vi "Poll Syringe-Line Valve Control.vi"(8 "error in (no error)":errorcluster, 11 "Syringe Line in":refnum<class "Syringe Line.lvclass">) -> ()   [LabVIEW 2015, in "cRIO-Carbondioxide.lvlib" / "CO2-Actor.lvlib" / "Syringe Line.lvclass"]
uses:
  Syringe Line.lvclass
  Syringe Line.lvclass/Syringe Line.ctl
  <vilib>/ActorFramework/Actor/Actor.lvclass/Actor.ctl
  <vilib>/ActorFramework/Message Enqueuer/Message Enqueuer.lvclass/Message Enqueuer.ctl
  Syringe Line Messages/Set Syringe Valve/Set Valve Msg/Set Syringe Valve Msg.lvclass/Set Syringe Valve Msg.ctl
  <vilib>/ActorFramework/Actor/Read Self Enqueuer.vi
  <vilib>/ActorFramework/Message Enqueuer/Enqueue.vi
  <vilib>/ActorFramework/Message Enqueuer/Init from Existing Queue.vi
  <vilib>/ActorFramework/Message Priority Queue/Priority Enqueue.vi
  <vilib>/ActorFramework/Actor/Actor.lvclass
  <vilib>/ActorFramework/Message Enqueuer/Message Enqueuer.lvclass
  Syringe Line Messages/Set Syringe Valve/Set Valve Msg/Set Syringe Valve Msg.lvclass
  cRIO-CO2/cRIO-CO2.lvclass
  CO2 Actor/CO2 Actor.lvclass
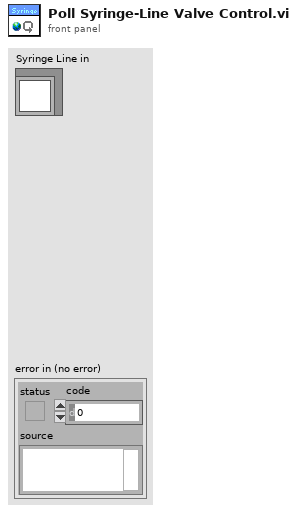
[diagram p1: front panel]
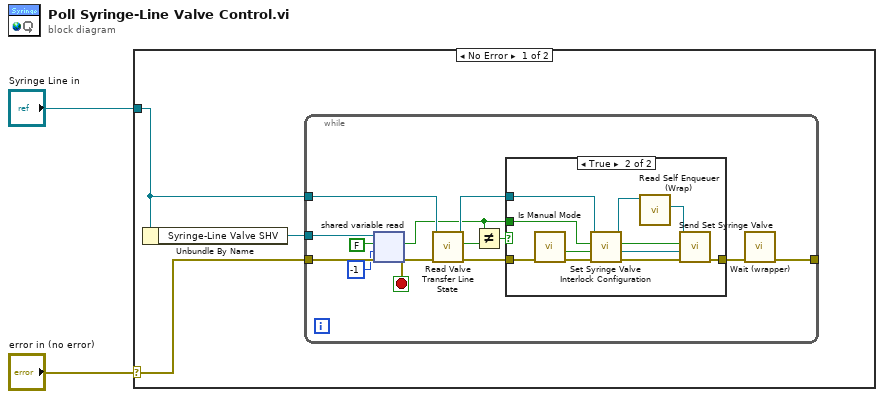
[diagram p0: block diagram]
diagram:
  n1 = case shown="No Error" "error in (no error)" {
    selector: "error in (no error)" -> [w3 _]
    tunnel: "Syringe Line in" -> [w4 _]
    frame No Error {
      n2 = Unbundle By Name(w4) -> ("Syringe-Line Valve SHV"=w5:refnum<k21>)
      n3 = while {
        tunnel: w5 -> [w18]
        tunnel: w3 -> [w17]
        tunnel: w4 -> [w11]
        tunnel: [w6] -> _
        stop <- w13 stop-if-true
        n4 = shared-variable-read(w18, w17, FALSE, -1 ("timeout ms")) -> (w13:errorcluster, w7:bool)  [unwired: 3 out]
        n5 = call "Read Valve Transfer Line State.vi"("error in (no error)"=w13, "Syringe Line in"=w11) -> ("error out"=w12:errorcluster, "Open?"=w9:bool, "Syringe Line out"=w10:refnum<class "Syringe Line.lvclass">)  [unwired: 6 in, 1 out]
        n6 = Not Equal?(x=w7, y=w9) -> (x != y?=w8:bool)
        n7 = case shown="True" w8 {
          tunnel: w7 -> [_ w28]
          tunnel: [w19 w22] -> w14
          tunnel: w12 -> [w19 w21]
          tunnel: w10 -> [_ w20]
          frame False {
          }
          frame True {
            n8 = call "Is Manual Mode.vi"("error in (no error)"=w21) -> ("error out"=w30:errorcluster, "Manual Mode?"=w29:bool)  [unwired: 9 in]
            n9 = call "Set Syringe Valve Interlock Configuration.vi"("error in (no error)"=w30, "Manual Mode (False)"=w29, "Open? (False)"=w28, "Syringe Line in"=w20) -> ("error out"=w27:errorcluster, "Interlock Chain"=w26:refnum<class "Interlock Chain.lvclass">, "Open? (False)"=w25:bool, "Syringe Line out"=w24:refnum<class "Syringe Line.lvclass">)  [unwired: 4 in]
            n10 = call "Read Self Enqueuer (Wrap).vi"("CO2 Actor in"=w24) -> ("Actor Framework:Message Enqueuer"=w23:refnum<class "Message Enqueuer.lvclass">)  [unwired: 9 in, 1 out]
            n11 = call "Send Set Syringe Valve.vi"("error in (no error)"=w27, "Interlock Chain.lvclass"=w26, "Open? (False)"=w25, "Message Enqueuer"=w23) -> ("error out"=w22:errorcluster)  [unwired: 6 in, 1 out]
          }
        }
        n12 = call "Wait (wrapper).vi"("error in (no error)"=w14) -> ("error out"=w6:errorcluster)  [unwired: 10 in]
      }
    }
    frame Error {
    }
  }
